vi "ACT_Loop.vi"() -> ()   [LabVIEW 2023, in "Pivot FX_ACT.lvlib"]
uses:
  Pivot FX_ACT.lvlib
  RoboRIO Utilities/Global_STOP.vi
  ENUM_ACT_Action.ctl
  ENUM_ACT_State.ctl
  Global_CMD_ACT_Data In.vi
  Global_ACT_Data Out.vi
  Cluster_CMD_ACT_Data.ctl
  <vilib>/Rock Robotics/WPI/MotorControl/WPI_MotorControlType.ctl
  <vilib>/Rock Robotics/SystemInterfaces/DIO/FPGA_DIOPWMChannel.ctl
  <vilib>/Rock Robotics/WPI/PWM/WPI_PWMDeadband.ctl
  <vilib>/Rock Robotics/SystemInterfaces/DIO/FPGA_DIOChannel.ctl
  <vilib>/Rock Robotics/WPI/MotorControl/WPI_MotorControlDeviceRef.ctl
  Shared Code/TypeDefs/Cluser_CAN Data.ctl
  <vilib>/Rock Robotics/WPI/ThirdParty/Phoenix-LabVIEW/Motor Controller/Controls/CTRE_Phoenix_MotorControl_NeutralMode.ctl
  Shared Code/TypeDefs/Cluster_FWD  REV Values.ctl
  Shared Code/TypeDefs/Cluster_PID Gains.ctl
  Shared Code/TypeDefs/Cluster_FX Motion Magic Parameters.ctl
  <vilib>/Rock Robotics/WPI/ThirdParty/Phoenix-LabVIEW/Motor Controller/Controls/CTRE_Phoenix_MotorControl_LimitSwitchNormal.ctl
  Shared Code/TypeDefs/Cluser_Hard Limits.ctl
  Shared Code/TypeDefs/Cluser_Enable-Value I32.ctl
  Shared Code/TypeDefs/Cluser_Config_Soft Limits.ctl
  Shared Code/TypeDefs/Cluser_FX Config_Limit Travel.ctl
  Cluster_Config HW Values.ctl
  b5508d6c-c1cc-4273-80c5-2077d34e1483.vi
  5f725c2a-0ce1-4524-8967-e83b15fdce90.vi
  <vilib>/Rock Robotics/WPI/ThirdParty/Phoenix-LabVIEW/Motor Controller/Controls/CTRE_Phoenix_MotorControl_ControlMode.ctl
  Shared Code/TypeDefs/Cluster_FX CloseLoop Values.ctl
  Shared Code/TypeDefs/Cluster_FX Current Values.ctl
  Cluster_HW Output Values.ctl
  ENUM_CMD_Mode Select.ctl
  4f1f8321-3dc8-4b28-8619-20673fc77ec2.vi
  Cluster_SW Output Data.ctl
  Cluster_Config SW Values.ctl
  36677ea0-a1a5-47a3-bc56-4475cb7c281e.vi
  573e44c0-11f4-4bd9-ad56-904ec25dba75.vi
  e7494af9-f670-4352-9dfa-ae6ce50709ea.vi
  6201c2b1-dcd8-4430-86f1-9b4ee56c7753.vi
  Shared Code/TypeDefs/Cluser_FX Config_Current Limits.ctl
  Shared Code/TypeDefs/Cluster_FX SLOT PID Config.ctl
  <vilib>/Rock Robotics/WPI/ThirdParty/Phoenix-LabVIEW/Motor Controller/Controls/CTRE_Phoenix_MotorControl_TalonFXInvertType.ctl
  Shared Code/TypeDefs/Cluster_Config FX Motor Output.ctl
  Shared Code/TypeDefs/ENUM_Pivot Arm Position Select.ctl
  Shared Code/TypeDefs/Cluster_Pivot Arm Position Table.ctl
  Shared Code/TypeDefs/Cluster_FX Limit Switchs.ctl
  Shared Code/TypeDefs/Cluster_FX Voltage Values.ctl
  Shared Code/TypeDefs/Cluster_FX Sensor Values.ctl
panel:
  out "STATE":T1
  in  "CMD Override":T2(tab)
  in  "Enable 1":bool
  in  "Percent Out":dbl(slide) scale=-1.0..1.0
  in  "Enable 2":bool
  in  "Position Counts":dbl
  in  "Enable 3":bool
  in  "Position Select":T3
  out "Current Time":timestamp
  in  "SW Config":T4={"Ver"=0, "Pivot Arm Position Table"={"Full Back"=0.0, "Full Forward"=140000.0, "Amp Score"=138000.0, "Pivot Arm Load"=17100.0, "Vertical"=72600.0, "Trap Score"=140000.0}}
  out "SW Output":T6
  out "Sensor Read time":dbl format="%.3g"
  out "HW Sensors":T7
  in  "Read Saved Config":bool
  in  "Update Config":bool
  in  "HW Config":T13 {"CL"."Gains"."F" format="%#.8f"; "CL"."Gains"."D" format="%#.8f"; "CL"."Gains"."I" format="%#.8f"; "CL"."Gains"."P" format="%#.8f"; "Output"."Min"."REV" format="%.2f"; "Output"."Min"."FWD" format="%.2f"; "Output"."Max"."REV" format="%.2f"; "Output"."Max"."FWD" format="%.2f"; "TravelLimits"."Soft"."REV"."Counts" format="%#.0f"; "TravelLimits"."Soft"."FWD"."Counts" format="%#.0f"}
  out "CMD":T28
  out "Cycle Time (S)":dbl format="%.3g"
  # "Teleop - Auto"
  # "STOP"
  # "Tune Output\nto 1023 Max"
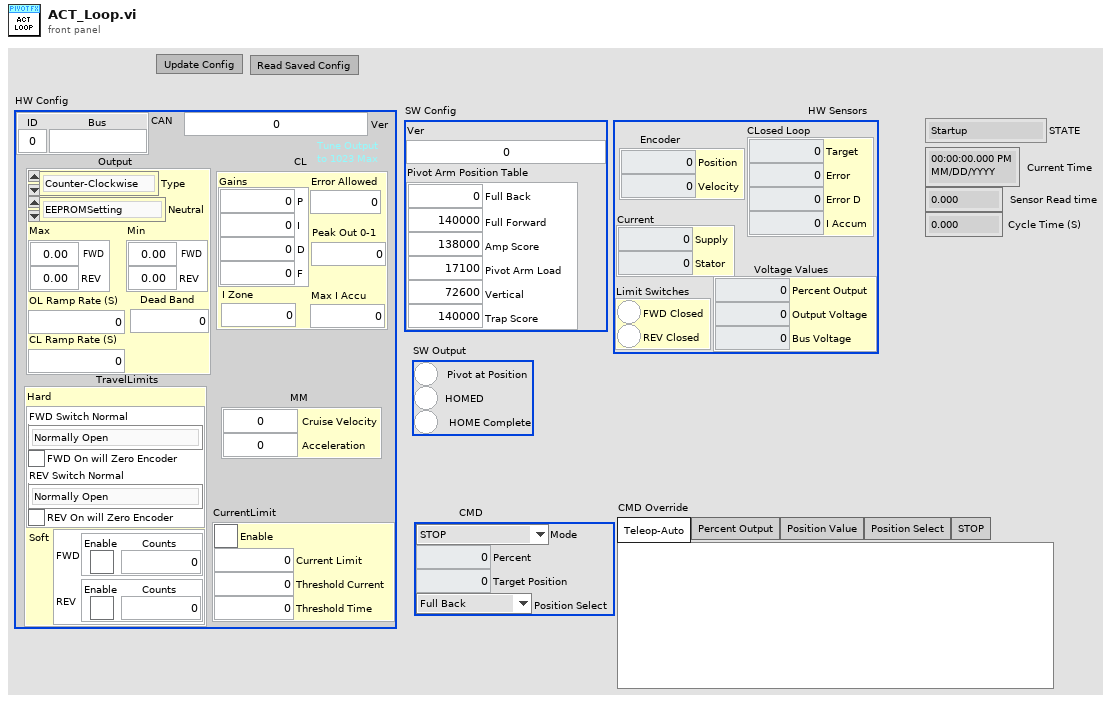
[diagram p1: front panel]
types:
  T1 = typedef "Pivot FX_ACT.lvlib/ENUM_ACT_State.ctl" = enum16{"Startup", "Configuring", "Homming", "Stopping", "Moving Percent Out", "Moving to Position", "Shutdown"}
  T2 = enum32{"Teleop-Auto", "Percent Output", "Position Value", "Position Select", "STOP"}
  T3 = typedef "ENUM_Pivot Arm Position Select.ctl" = enum16{"Full Back", "Full Forward", "Amp Score", "Pivot Arm Load", "Vertical", "Trap Score"}
  T4 = typedef "Pivot FX_ACT.lvlib/Cluster_Config SW Values.ctl" = cluster{"Ver":u64, "Pivot Arm Position Table":T5}
  T5 = typedef "Cluster_Pivot Arm Position Table.ctl" = cluster{"Full Back":dbl, "Full Forward":dbl, "Amp Score":dbl, "Pivot Arm Load":dbl, "Vertical":dbl, "Trap Score":dbl}
  T6 = typedef "Pivot FX_ACT.lvlib/Cluster_SW Output Data.ctl" = cluster{"Pivot at Position":bool, "HOMED":bool, "HOME Complete":bool}
  T7 = typedef "Pivot FX_ACT.lvlib/Cluster_HW Output Values.ctl" = cluster{"CLosed Loop":T8, "Current":T9, "Limit Switches":T10, "Voltage Values":T11, "Encoder ":T12}
  T8 = typedef "Cluster_FX CloseLoop Values.ctl" = cluster{"Target":dbl, "Error":i32, "Error D":dbl, "I Accum":dbl}
  T9 = typedef "Cluster_FX Current Values.ctl" = cluster{"Supply":dbl, "Stator":dbl}
  T10 = typedef "Cluster_FX Limit Switchs.ctl" = cluster{"FWD Closed":bool, "REV Closed":bool}
  T11 = typedef "Cluster_FX Voltage Values.ctl" = cluster{"Percent Output":dbl, "Output Voltage":dbl, "Bus Voltage":dbl}
  T12 = typedef "Cluster_FX Sensor Values.ctl" = cluster{"Position":i32, "Velocity":i32}
  T13 = typedef "Pivot FX_ACT.lvlib/Cluster_Config HW Values.ctl" = cluster{"Ver":u64, "CAN":T14, "Output":T15, "CL":T19, "MM":T21, "TravelLimits":T22, "CurrentLimit":T27}
  T14 = typedef "Cluser_CAN Data.ctl" = cluster{"ID":u8, "Bus":string}
  T15 = typedef "Cluster_Config FX Motor Output.ctl" = cluster{"Type":T16, "Neutral":T17, "Max":T18, "Min":T18, "OL Ramp Rate (S)":dbl, "Dead Band":dbl, "CL Ramp Rate (S)":dbl}
  T16 = typedef "CTRE_Phoenix_MotorControl_TalonFXInvertType.ctl" = enum16{"Counter-Clockwise", "Clockwise"}
  T17 = typedef "CTRE_Phoenix_MotorControl_NeutralMode.ctl" = enum8{"EEPROMSetting", "Override to Coast", "Override to Brake"}
  T18 = typedef "Cluster_FWD  REV Values.ctl" = cluster{"FWD":dbl, "REV":dbl}
  T19 = typedef "Cluster_FX SLOT PID Config.ctl" = cluster{"Gains":T20, "Error Allowed":dbl, "I Zone":dbl, "Peak Out 0-1":dbl, "Max I Accu":dbl}
  T20 = typedef "Cluster_PID Gains.ctl" = cluster{"P":dbl, "I":dbl, "D":dbl, "F":dbl}
  T21 = typedef "Cluster_FX Motion Magic Parameters.ctl" = cluster{"Cruise Velocity":i32, "Acceleration":i32}
  T22 = typedef "Cluser_FX Config_Limit Travel.ctl" = cluster{"Hard":T23, "Soft":T25}
  T23 = typedef "Cluser_Hard Limits.ctl" = cluster{"FWD Switch Normal":T24, "FWD On will Zero Encoder ":bool, "REV Switch Normal":T24, "REV On will Zero Encoder ":bool}
  T24 = typedef "CTRE_Phoenix_MotorControl_LimitSwitchNormal.ctl" = enum16{"Normally Open", "Normally Closed", "Disabled"}
  T25 = typedef "Cluser_Config_Soft Limits.ctl" = cluster{"FWD":T26, "REV":T26}
  T26 = typedef "Cluser_Enable-Value I32.ctl" = cluster{"Enable":bool, "Counts":i32}
  T27 = typedef "Cluser_FX Config_Current Limits.ctl" = cluster{"Enable":bool, "Current Limit":dbl, "Threshold Current":dbl, "Threshold Time":dbl}
  T28 = typedef "Pivot FX_ACT.lvlib/Cluster_CMD_ACT_Data.ctl" = cluster{"Mode":T29, "Percent":dbl, "Target Position":dbl, "Position Select":T3}
  T29 = typedef "Pivot FX_ACT.lvlib/ENUM_CMD_Mode Select.ctl" = enum16{"STOP", "PercentOut", "Positon Value", "Position Select"}
  T30 = typedef "CTRE_Phoenix_MotorControl_ControlMode.ctl" = u16
  T31 = typedef "WPI_MotorControlDeviceRef.ctl" = cluster{"DeviceStatus":errorcluster, "Type":T32, "PWM":cluster{"PWM Channel":T33, "DeadBand":T34}, "CAN":cluster{"Device Number":u8, "SetOutput VI Ref":variant, "GetOutput VI Ref":variant, "Enable VI Ref":variant, "Disable VI Ref":variant, "Data":variant}, "Invert":bool, "DIO PWM":cluster{"PWM \"Enable\" Channel":T33, "DIOChannel":T35, "PWM Rate":dbl}}
  T32 = typedef "WPI_MotorControlType.ctl" = enum16{"PWM", "CAN", "DIO PWM"}
  T33 = typedef "FPGA_DIOPWMChannel.ctl" = enum8{"PWM 0", "PWM 1", "PWM 2", "PWM 3", "PWM 4", "PWM 5", "PWM 6", "PWM 7", "PWM 8", "PWM 9", "PWM MXP 0", "PWM MXP 1", "PWM MXP 2", "PWM MXP 3", "PWM MXP 4", "PWM MXP 5", "PWM MXP 6", "PWM MXP 7", "PWM MXP 8", "PWM MXP 9", "Invalid"}
  T34 = typedef "WPI_PWMDeadband.ctl" = cluster{"Name":string, "maxPositivePwm":i32, "minPositivePwm":i32, "centerPwm":i32, "maxNegativePwm":i32, "minNegativePwm":i32, "angularRange":u16}
  T35 = typedef "FPGA_DIOChannel.ctl" = enum8{"DIO 0", "DIO 1", "DIO 2", "DIO 3", "DIO 4", "DIO 5", "DIO 6", "DIO 7", "DIO 8", "DIO 9", "DIO MXP 0", "DIO MXP 1", "DIO MXP 2", "DIO MXP 3", "DIO MXP 4", "DIO MXP 5", "DIO MXP 6", "DIO MXP 7", "DIO MXP 8", "DIO MXP 9", "DIO MXP 10", "DIO MXP 11", "DIO MXP 12", "DIO MXP 13", "DIO MXP 14", "DIO MXP 15", "SPI Port CS1", "SPI Port CS2", "SPI Port CS3", "SPI Port MISO", "SPI Port MOSI", "Invalid"}
  T36 = cluster{"Team Files Folder":path, "FX Ref":T31, "State":T1, "Previous State":T1, "Current Time":timestamp, "Previous Time":timestamp, "Start Time":timestamp, "Target Time (ms)":u32, "Cycle Time(S)":dbl, "Update Display":bool, "ACT Input":T28, "HW Config":T13, "SW Config":T4, "Max # Of Config Tries":i32, "HW Out":T7, "SW Out":T6, "CAN Timeout":u32, "FX Mode":T30, "FX Set Value":dbl}
  T37 = typedef "Pivot FX_ACT.lvlib/ENUM_ACT_Action.ctl" = enum16{"No Action", "Reset Time", "Reset All", "Config HW File Read", "Config HW File Save", "Config SW File Read", "Config SW File Save", "Config From FP", "Config HW Get", "Config HW Set", "Open HW Only", "Control FX Stop", "Control FX Percent Out", "Control FX Position Value", "Control FX Position Select", "Control FX GoTo HOME", "Encoder Set to Zero"}
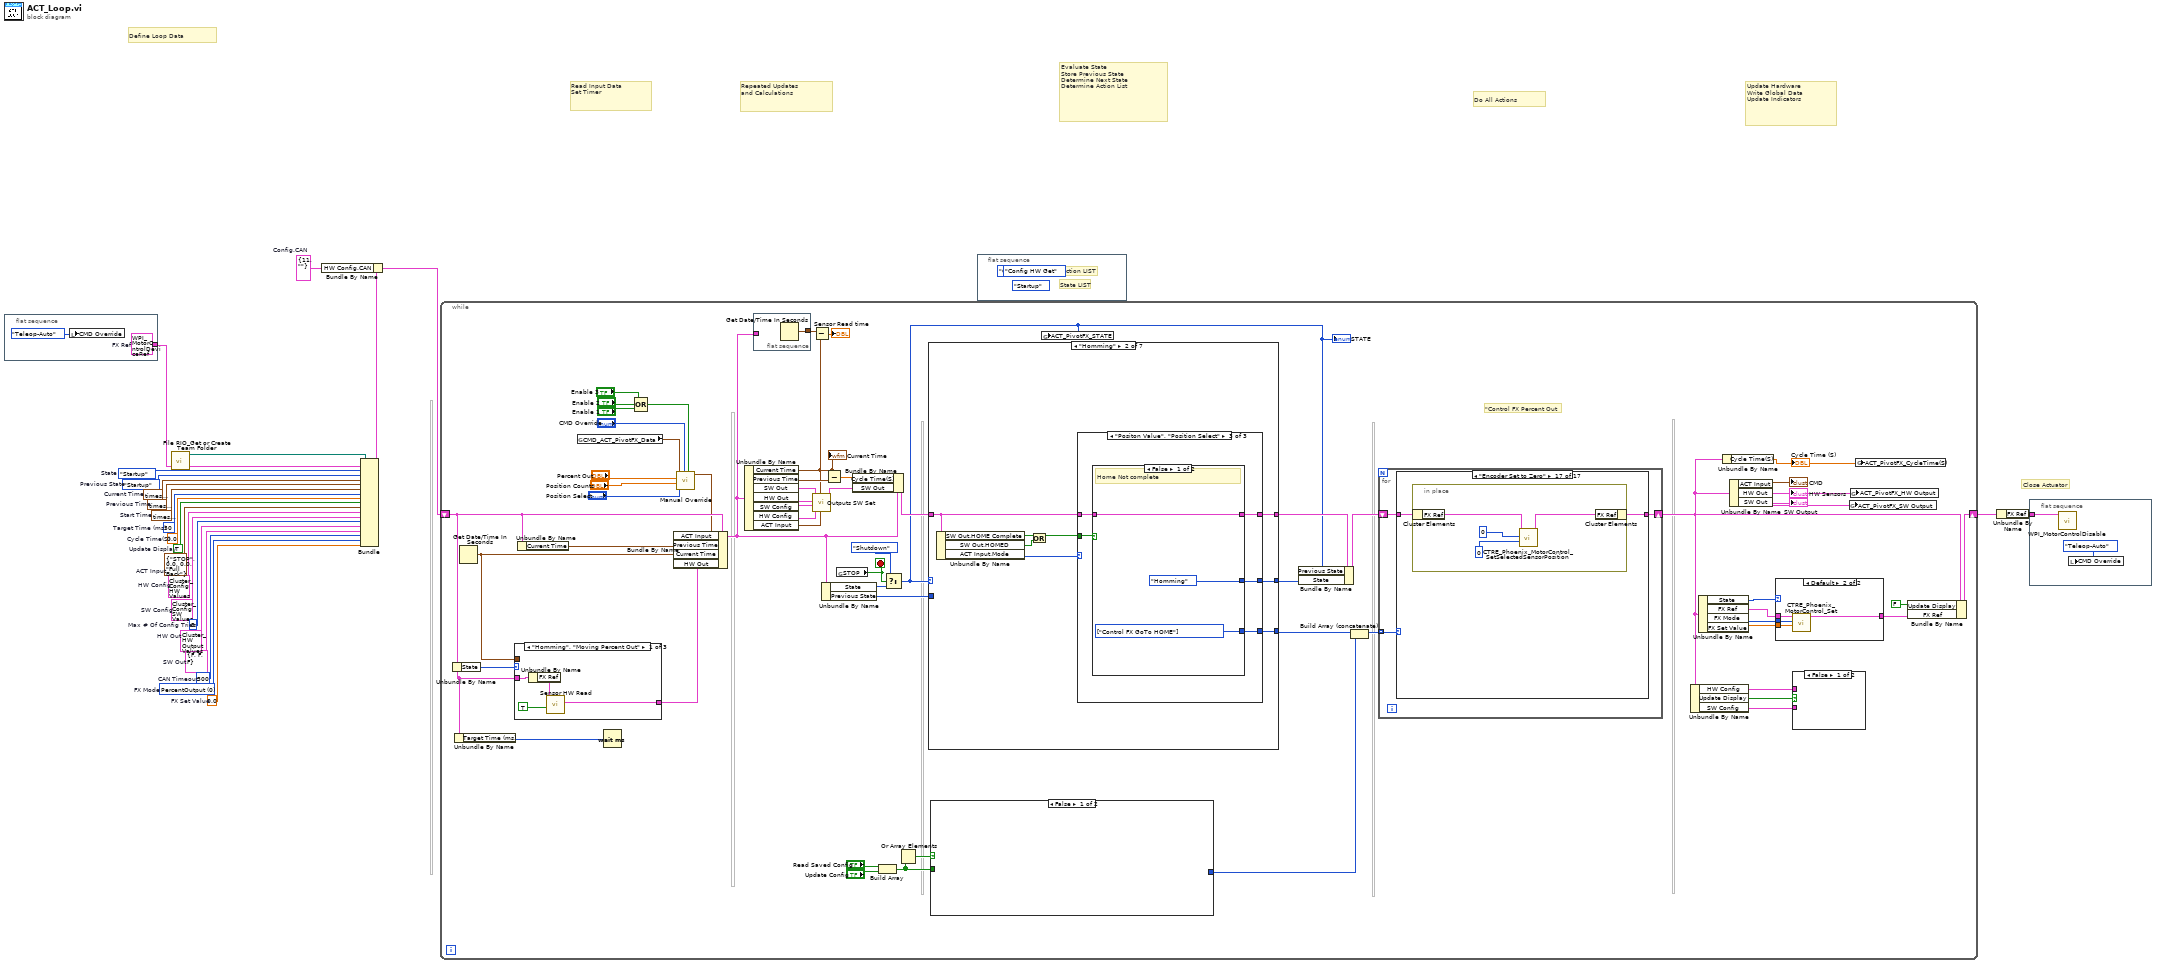
[diagram p0: block diagram]
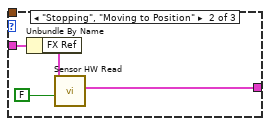
[diagram p2: hidden frame]
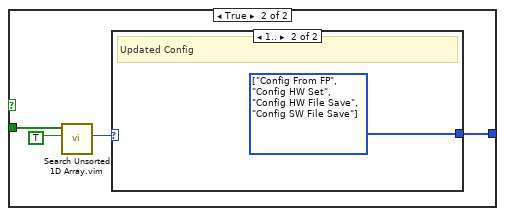
[diagram p4: hidden frame]
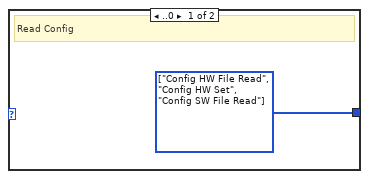
[diagram p5: hidden frame]
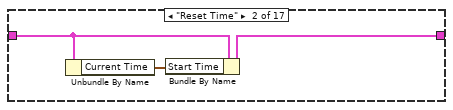
[diagram p7: hidden frame]
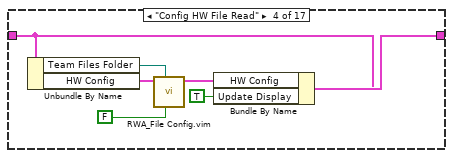
[diagram p9: hidden frame]
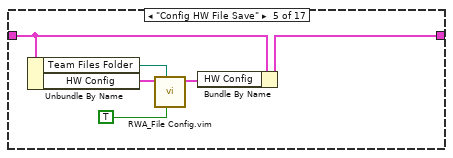
[diagram p10: hidden frame]
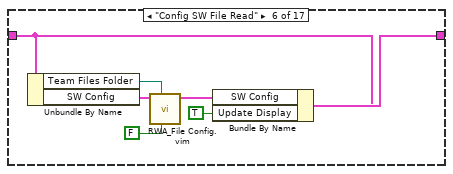
[diagram p11: hidden frame]
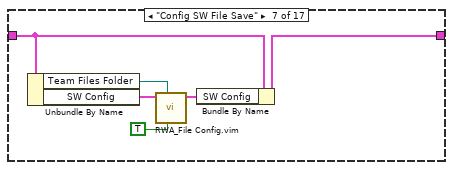
[diagram p12: hidden frame]
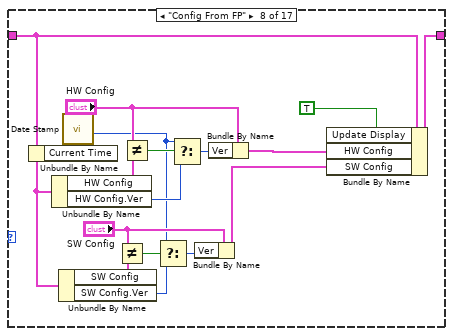
[diagram p13: hidden frame]
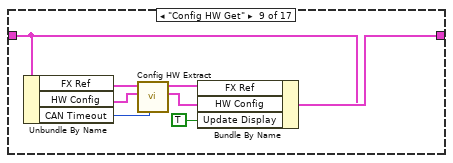
[diagram p14: hidden frame]
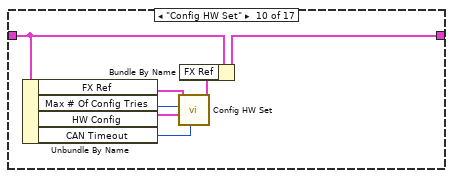
[diagram p15: hidden frame]
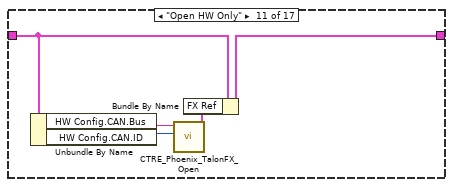
[diagram p16: hidden frame]
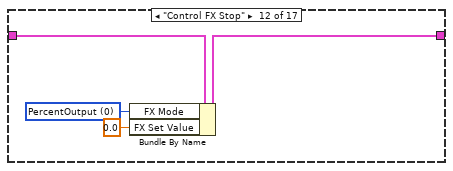
[diagram p17: hidden frame]
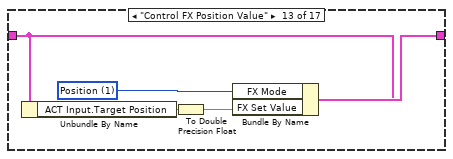
[diagram p18: hidden frame]
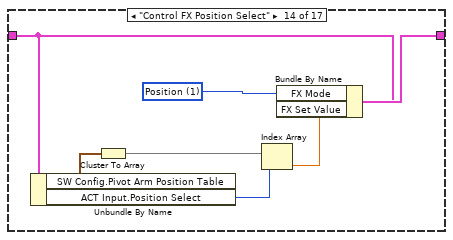
[diagram p19: hidden frame]
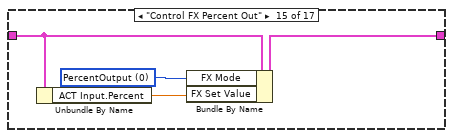
[diagram p20: hidden frame]
diagram:
  w1 = T4 {"Ver"=0, "Pivot Arm Position Table"={"Full Back"=0.0, "Full Forward"=140000.0, "Amp Score"=138473.0, "Pivot Arm Load"=17141.0, "Vertical"=72668.0, "Trap Score"=140000.0}}  # SW Config
  w10 = T13 {"Ver"=0, "CAN"={"ID"=0, "Bus"=""}, "Output"={"Type"=enum."Counter-Clockwise", "Neutral"=enum."EEPROMSetting", "Max"={"FWD"=0.0, "REV"=0.0}, "Min"={"FWD"=0.0, "REV"=0.0}, "OL Ramp Rate (S)"=0.0, "Dead Band"=0.0, "CL Ramp Rate (S)"=0.0}, "CL"={"Gains"={"P"=0.0, "I"=0.0, "D"=0.0, "F"=0.0}, "Error Allowed"=0.0, "I Zone"=0.0, "Peak Out 0-1"=0.0, "Max I Accu"=0.0}, "MM"={"Cruise Velocity"=0, "Acceleration"=0}, "TravelLimits"={"Hard"={"FWD Switch Normal"=enum."Normally Open", "FWD On will Zero Encoder "=FALSE, "REV Switch Normal"=enum."Normally Open", "REV On will Zero Encoder "=FALSE}, "Soft"={"FWD"={"Enable"=FALSE, "Counts"=0}, "REV"={"Enable"=FALSE, "Counts"=0}}}, "CurrentLimit"={"Enable"=FALSE, "Current Limit"=0.0, "Threshold Current"=0.0, "Threshold Time"=0.0}}  # HW Config
  w8 = T6 {"Pivot at Position"=FALSE, "HOMED"=FALSE, "HOME Complete"=FALSE}  # SW Out
  w9 = T7 {"CLosed Loop"={"Target"=0.0, "Error"=0, "Error D"=0.0, "I Accum"=0.0}, "Current"={"Supply"=0.0, "Stator"=0.0}, "Limit Switches"={"FWD Closed"=FALSE, "REV Closed"=FALSE}, "Voltage Values"={"Percent Output"=0.0, "Output Voltage"=0.0, "Bus Voltage"=0.0}, "Encoder "={"Position"=0, "Velocity"=0}}  # HW Out
  w4 = 0.0  # FX Set Value
  w5 = T30 0 items=["PercentOutput"=0, "Position"=1, "Velocity"=2, "Current"=3, "Follower"=5, "MotionProfile"=6, "MotionMagic"=7, "MotionProfileArc"=10, "Disabled"=15]  # FX Mode
  w3 = u32 300  # CAN Timeout
  w2 = 3  # Max # Of Config Tries
  w12 = TRUE  # Update Display
  w13 = T14 {"ID"=11, "Bus"=""}  # Config.CAN
  w18 = 0.0  # Cycle Time(S)
  w19 = ENUM_ACT_State."Startup"  # Previous State
  w20 = timestamp(0 s since 1904-01-01)  # Previous Time
  w21 = u32 50  # Target Time (ms)
  w7 = T28 {"Mode"=enum."STOP", "Percent"=0.0, "Target Position"=0.0, "Position Select"=enum."Full Back"}  # ACT Input
  w22 = timestamp(0 s since 1904-01-01)  # Start Time
  w23 = timestamp(0 s since 1904-01-01)  # Current Time
  w24 = ENUM_ACT_State."Startup"  # State
  # "Close Actuator"
  # "Define Loop Data"
  # "Repeated Updates\nand Calculations"
  # "Read Input Data\nSet Timer"
  # "Evaluate State\nStore Previous State\nDetermine Next State\nDetermine Action List"
  # "Do All Actions"
  # "Update Hardware\nWrite Global Data\nUpdate Indicators"
  n1 = flat-sequence {
    tunnel: [w26] -> w14
    frame #0 {
      w26 = T31 {"DeviceStatus"={"status"=FALSE, "code"=0, "source"=""}, "Type"=enum."PWM", "PWM"={"PWM Channel"=enum."PWM 1", "DeadBand"={"Name"="", "maxPositivePwm"=0, "minPositivePwm"=0, "centerPwm"=0, "maxNegativePwm"=0, "minNegativePwm"=0, "angularRange"=0}}, "CAN"={"Device Number"=0, "SetOutput VI Ref"=variant(enum8{"Percent VBus", "Current", "Speed", "Position", "Voltage"} enum."Percent VBus"), "GetOutput VI Ref"=variant(refnum<k1> refnum), "Enable VI Ref"=variant(dbl 12.0), "Disable VI Ref"=variant(enum8{"Percent VBus", "Speed", "Position", "Slave", "Unchanged / Invalid", "Voltage Compensation", "Current", "Motion Profile"} enum."Percent VBus"), "Data"=variant}, "Invert"=FALSE, "DIO PWM"={"PWM \"Enable\" Channel"=enum."Invalid", "DIOChannel"=enum."Invalid", "PWM Rate"=0.0}}  # FX Ref
      n2 = local write "CMD Override"(T2."Teleop-Auto" ("CMD Override")) -> ()
    }
  }
  n3 = call "File RIO_Get or Create Team Folder.vi"() -> ("Team Files Folder"=w6:path)  [unwired: 10 in, 1 out]
  n4 = Bundle("Team Files Folder"=w6, "FX Ref"=w14, "State"=w24, "Previous State"=w19, "Current Time"=w23, "Previous Time"=w20, "Start Time"=w22, "Target Time (ms)"=w21, "Cycle Time(S)"=w18, "Update Display"=w12, "ACT Input"=w7, "HW Config"=w10, "SW Config"=w1, "Max # Of Config Tries"=w2, "HW Out"=w9, "SW Out"=w8, "CAN Timeout"=w3, "FX Mode"=w5, "FX Set Value"=w4) -> (w16:T36)  [unwired: 1 in]
  n5 = Bundle By Name(cluster=w16, "HW Config.CAN"=w13) -> (w15:T36)
  n6 = while {
    shift-right: [w69] -> w17
    shift-left: w15 -> [w39]
    stop <- w82 stop-if-true
    # "\"Control FX Percent Out"
    n7 = Unbundle By Name(w39) -> ("State"=w59:T1)
    n8 = Unbundle By Name(w39) -> ("Target Time (ms)"=w79:u32)
    n9 = Get Date/Time In Seconds() -> (seconds since 1Jan1904=w55:timestamp)
    n10 = case shown="\"Homming\", \"Moving Percent Out\"" w59 {
      tunnel: w39 -> [w90 w94 _]
      tunnel: w55 -> [_ _ _]
      tunnel: [w87 w91 _] -> w40
      frame "Homming", "Moving Percent Out" {
        n11 = Unbundle By Name(w90) -> ("FX Ref"=w89:T31)
        n12 = call "Sensor HW Read.vi"("Read Closed Loop"=TRUE, "Ref"=w89) -> ("Sensor Values Out"=w87:T7)  [unwired: 7 in, 2 out]
      }
      frame "Stopping", "Moving to Position" {
        n13 = Unbundle By Name(w94) -> ("FX Ref"=w93:T31)
        n14 = call "Sensor HW Read.vi"("Read Closed Loop"=FALSE, "Ref"=w93) -> ("Sensor Values Out"=w91:T7)  [unwired: 7 in, 2 out]
      }
      frame "Startup", "Configuring", "Shutdown" {
      }
    }
    n15 = Unbundle By Name(w39) -> ("Current Time"=w78:timestamp)
    n16 = global read "Global_CMD_ACT_Data In.vi" "CMD_ACT_PivotFX_Data"() -> (w36:T28)
    n17 = Wait (ms)(milliseconds to wait=w79) -> ()  [unwired: 1 out]
    n18 = Compound Arithmetic op=OR("Enable 3", "Enable 2", "Enable 1") -> (w32:bool)
    n19 = call "Manual Override.vi"("Enable"=w32, "CMD Override"="CMD Override", "Pivot Position Select"="Position Select", "Position Data"="Position Counts", "Percent Out Data"="Percent Out", "Auto CMD"=w36) -> ("OverRide Command Out"=w38:T28)  [unwired: 5 in]
    n20 = Bundle By Name(cluster=w39, "ACT Input"=w38, "Previous Time"=w78, "Current Time"=w55, "HW Out"=w40) -> (w41:T36)
    n21 = Unbundle By Name(w41) -> ("Current Time"=w45:timestamp, "Previous Time"=w76:timestamp, "SW Out"=w48:T6, "HW Out"=w46:T7, "SW Config"=w44:T4, "HW Config"=w43:T13, "ACT Input"=w27:T28)
    "Current Time" <- w45
    n22 = flat-sequence {
      tunnel: [w86] -> w57
      tunnel: w41 -> [_]
      frame #0 {
        n23 = Get Date/Time In Seconds() -> (seconds since 1Jan1904=w86:timestamp)
      }
    }
    n24 = call "Outputs SW Set.vi"("CMD_ACT_Tempplate Data"=w27, "Current Time"=w45, "HW Config"=w43, "SW Config"=w44, "Sensor Values"=w46, "SW Output"=w48) -> ("SW Output Out"=w47:T6)  [unwired: 5 in]
    n25 = Subtract(x=w57, y=w45) -> (x-y=→"Sensor Read time":dbl)
    n26 = Unbundle By Name(w41) -> ("State"=w80:T1, "Previous State"=w77:T1)
    n27 = Subtract(x=w45, y=w76) -> (x-y=w74:dbl)
    n28 = global read "Global_STOP.vi" "STOP"() -> (w82:bool)
    n29 = Bundle By Name(cluster=w41, "Cycle Time(S)"=w74, "SW Out"=w47) -> (w75:T36)
    n30 = Build Array("Read Saved Config", "Update Config") -> (w51:bool[])
    n31 = Select(t=ENUM_ACT_State."Shutdown" ("State"), s=w82, f=w80) -> (s? t:f=w37:T1)
    "STATE" <- w37
    n32 = Or Array Elements(Boolean array=w51) -> (logical OR=w52:bool)
    n33 = case shown="\"Homming\"" w37 {
      selector: w37 -> [_ _ w253 w273 _ _ _]
      tunnel: w75 -> [w207 w232 w254 w274 w301 w304 w309]
      tunnel: [w210 w231 w255 w275 w301 w304 w308] -> w84
      tunnel: [w209 w229 w257 w277 ENUM_ACT_State."Shutdown" ("State") ENUM_ACT_State."Configuring" ("State") w307] -> w83
      tunnel: [w208 w230 w252 w271 w299 w303 w305] -> w73
      tunnel: w77 -> [_ _ _ _ _ _ _]
      frame "Configuring" {
        n34 = Unbundle By Name(w207) -> ("SW Config"=w205:T4)
        n35 = Unbundle By Name(w207) -> ("Team Files Folder"=w204:path, "HW Config"=w212:T13)
        n36 = call "Config_Build Name.vim"("Config First Name"=w212) -> ("Cfg file"=w214:string)  [unwired: 9 in, 1 out]
        n37 = call "Config_Build Name.vim"("Config First Name"=w205) -> ("Cfg file"=w206:string)  [unwired: 9 in, 1 out]
        n38 = Build Path(base path=w204, name or relative path=w206) -> (appended path=w203:path)
        n39 = Build Path(base path=w204, name or relative path=w214) -> (appended path=w213:path)
        n40 = call <vilib>:"Check if File or Folder Exists.vi"("path"=w203) -> ("file or folder exists?"=w202:bool)  [unwired: 8 in, 2 out]
        n41 = call <vilib>:"Check if File or Folder Exists.vi"("path"=w213) -> ("file or folder exists?"=w211:bool)  [unwired: 8 in, 2 out]
        n42 = case shown="True" w211 {
          tunnel: w207 -> [w217 w221]
          tunnel: [w217 w221] -> w210
          tunnel: [ENUM_ACT_State."Configuring" ("State") w220] -> w209
          tunnel: [w215 w219] -> w208
          tunnel: w202 -> [_ w218]
          frame False {
            w215 = T37[] [enum."Open HW Only", enum."Config HW Get", enum."Config HW File Save"] items=["No Action", "Reset Time", "Reset All", "Config HW File Read", "Config HW File Save", "Config SW File Read", "Config SW File Save", "Config From FP", "Config HW Get", "Config HW Set", "Open HW Only", "Control FX Stop", "Control FX Percent Out", "Control FX Position Value", "Control FX Position Select", "Control FX GoTo HOME", "Encoder Set to Zero"] ("Actions")
            # "HW Config File Not Found"
          }
          frame True {
            # "HW Config File Found"
            n43 = case shown="True" w218 {
              tunnel: [ENUM_ACT_State."Configuring" ("State") ENUM_ACT_State."Stopping" ("State")] -> w220
              tunnel: [w222 w224] -> w219
              frame False {
                w222 = T37[] [enum."Config SW File Save"] items=["No Action", "Reset Time", "Reset All", "Config HW File Read", "Config HW File Save", "Config SW File Read", "Config SW File Save", "Config From FP", "Config HW Get", "Config HW Set", "Open HW Only", "Control FX Stop", "Control FX Percent Out", "Control FX Position Value", "Control FX Position Select", "Control FX GoTo HOME", "Encoder Set to Zero"] ("Actions")
                # "SW Config File NOT Found"
              }
              frame True {
                w224 = T37[] [enum."Config HW File Read", enum."Config HW Set", enum."Config SW File Read", enum."Reset All", enum."Control FX Stop"] items=["No Action", "Reset Time", "Reset All", "Config HW File Read", "Config HW File Save", "Config SW File Read", "Config SW File Save", "Config From FP", "Config HW Get", "Config HW Set", "Open HW Only", "Control FX Stop", "Control FX Percent Out", "Control FX Position Value", "Control FX Position Select", "Control FX GoTo HOME", "Encoder Set to Zero"] ("Actions")
                # "SW Config File Found"
              }
            }
          }
        }
      }
      frame "Homming" {
        n44 = Unbundle By Name(w232) -> ("SW Out.HOME Complete"=w233:bool, "SW Out.HOMED"=w227:bool, "ACT Input.Mode"=w226:T29)
        n45 = Or(x=w233, y=w227) -> (x .or. y?=w228:bool)
        n46 = case shown="\"Positon Value\", \"Position Select\"" w226 {
          tunnel: w232 -> [w236 w239 w244]
          tunnel: [w236 w239 w243] -> w231
          tunnel: [w234 w237 w242] -> w230
          tunnel: [ENUM_ACT_State."Stopping" ("State") ENUM_ACT_State."Moving Percent Out" ("State") w241] -> w229
          tunnel: w228 -> [_ _ w240]
          frame "STOP" {
            w234 = T37[] [enum."Control FX Stop"] items=["No Action", "Reset Time", "Reset All", "Config HW File Read", "Config HW File Save", "Config SW File Read", "Config SW File Save", "Config From FP", "Config HW Get", "Config HW Set", "Open HW Only", "Control FX Stop", "Control FX Percent Out", "Control FX Position Value", "Control FX Position Select", "Control FX GoTo HOME", "Encoder Set to Zero"] ("Actions")
          }
          frame "PercentOut" {
            w237 = T37[] [enum."Control FX Stop"] items=["No Action", "Reset Time", "Reset All", "Config HW File Read", "Config HW File Save", "Config SW File Read", "Config SW File Save", "Config From FP", "Config HW Get", "Config HW Set", "Open HW Only", "Control FX Stop", "Control FX Percent Out", "Control FX Position Value", "Control FX Position Select", "Control FX GoTo HOME", "Encoder Set to Zero"] ("Actions")
          }
          frame "Positon Value", "Position Select" {
            n47 = case shown="False" w240 {
              tunnel: w244 -> [w247 w248]
              tunnel: [w247 w248] -> w243
              tunnel: [w245 w250] -> w242
              tunnel: [ENUM_ACT_State."Homming" ("State") ENUM_ACT_State."Stopping" ("State")] -> w241
              frame False {
                w245 = T37[] [enum."Control FX GoTo HOME"] items=["No Action", "Reset Time", "Reset All", "Config HW File Read", "Config HW File Save", "Config SW File Read", "Config SW File Save", "Config From FP", "Config HW Get", "Config HW Set", "Open HW Only", "Control FX Stop", "Control FX Percent Out", "Control FX Position Value", "Control FX Position Select", "Control FX GoTo HOME", "Encoder Set to Zero"] ("Actions")
                # "Home Not complete"
              }
              frame True {
                w250 = T37[] [enum."Control FX Stop", enum."Encoder Set to Zero"] items=["No Action", "Reset Time", "Reset All", "Config HW File Read", "Config HW File Save", "Config SW File Read", "Config SW File Save", "Config From FP", "Config HW Get", "Config HW Set", "Open HW Only", "Control FX Stop", "Control FX Percent Out", "Control FX Position Value", "Control FX Position Select", "Control FX GoTo HOME", "Encoder Set to Zero"] ("Actions")
                # "Home Complete"
              }
            }
          }
        }
      }
      frame "Moving Percent Out" {
        w251 = T37[] [enum."Control FX Stop"] items=["No Action", "Reset Time", "Reset All", "Config HW File Read", "Config HW File Save", "Config SW File Read", "Config SW File Save", "Config From FP", "Config HW Get", "Config HW Set", "Open HW Only", "Control FX Stop", "Control FX Percent Out", "Control FX Position Value", "Control FX Position Select", "Control FX GoTo HOME", "Encoder Set to Zero"] ("Actions")
        n48 = Unbundle By Name(w254) -> ("ACT Input.Mode"=w256:T29)
        n49 = case shown="\"Position Select\"" w256 {
          tunnel: [ENUM_ACT_State."Stopping" ("State") ENUM_ACT_State."Moving to Position" ("State") ENUM_ACT_State."Moving to Position" ("State") w268] -> w257
          tunnel: w254 -> [w260 w263 w266 w269]
          tunnel: [w260 w263 w266 w269] -> w255
          tunnel: w253 -> [_ _ _ w268]
          tunnel: [w258 w261 w264 w267] -> w252
          tunnel: w251 -> [w258 w261 w264 _]
          frame "STOP" {
          }
          frame "Positon Value" {
          }
          frame "Position Select" {
          }
          frame "PercentOut" {
            w267 = T37[] [enum."Control FX Percent Out"] items=["No Action", "Reset Time", "Reset All", "Config HW File Read", "Config HW File Save", "Config SW File Read", "Config SW File Save", "Config From FP", "Config HW Get", "Config HW Set", "Open HW Only", "Control FX Stop", "Control FX Percent Out", "Control FX Position Value", "Control FX Position Select", "Control FX GoTo HOME", "Encoder Set to Zero"] ("Actions")
          }
        }
      }
      frame "Moving to Position" {
        w272 = T37[] [enum."Control FX Stop"] items=["No Action", "Reset Time", "Reset All", "Config HW File Read", "Config HW File Save", "Config SW File Read", "Config SW File Save", "Config From FP", "Config HW Get", "Config HW Set", "Open HW Only", "Control FX Stop", "Control FX Percent Out", "Control FX Position Value", "Control FX Position Select", "Control FX GoTo HOME", "Encoder Set to Zero"] ("Actions")
        n50 = Unbundle By Name(w274) -> ("SW Out.HOME Complete"=w270:bool, "ACT Input.Mode"=w276:T29)
        n51 = case shown="True" w270 {
          tunnel: [ENUM_ACT_State."Homming" ("State") w286] -> w277
          tunnel: w276 -> [_ w285]
          tunnel: [w279 w284] -> w275
          tunnel: w274 -> [w279 w283]
          tunnel: w273 -> [_ w282]
          tunnel: w272 -> [_ w281]
          tunnel: [_ w280] -> w271
          frame False {
            # "Home Not Complete"
          }
          frame True {
            # "Home Complete"
            n52 = case shown="\"Positon Value\"" w285 {
              tunnel: [ENUM_ACT_State."Stopping" ("State") w290 w294 ENUM_ACT_State."Moving Percent Out" ("State")] -> w286
              tunnel: w283 -> [w289 w292 w293 w298]
              tunnel: [w289 w292 w293 w298] -> w284
              tunnel: w282 -> [_ w290 w294 _]
              tunnel: [w287 w291 w295 w296] -> w280
              tunnel: w281 -> [w287 _ _ w296]
              frame "STOP" {
              }
              frame "Positon Value" {
                w291 = T37[] [enum."Control FX Position Value"] items=["No Action", "Reset Time", "Reset All", "Config HW File Read", "Config HW File Save", "Config SW File Read", "Config SW File Save", "Config From FP", "Config HW Get", "Config HW Set", "Open HW Only", "Control FX Stop", "Control FX Percent Out", "Control FX Position Value", "Control FX Position Select", "Control FX GoTo HOME", "Encoder Set to Zero"] ("Actions")
              }
              frame "Position Select" {
                w295 = T37[] [enum."Control FX Position Select"] items=["No Action", "Reset Time", "Reset All", "Config HW File Read", "Config HW File Save", "Config SW File Read", "Config SW File Save", "Config From FP", "Config HW Get", "Config HW Set", "Open HW Only", "Control FX Stop", "Control FX Percent Out", "Control FX Position Value", "Control FX Position Select", "Control FX GoTo HOME", "Encoder Set to Zero"] ("Actions")
              }
              frame "PercentOut" {
              }
            }
          }
        }
      }
      frame "Shutdown" {
        w299 = T37[] [enum."Reset All"] items=["No Action", "Reset Time", "Reset All", "Config HW File Read", "Config HW File Save", "Config SW File Read", "Config SW File Save", "Config From FP", "Config HW Get", "Config HW Set", "Open HW Only", "Control FX Stop", "Control FX Percent Out", "Control FX Position Value", "Control FX Position Select", "Control FX GoTo HOME", "Encoder Set to Zero"] ("Actions")
      }
      frame "Startup" {
        w303 = T37[] [enum."Reset Time"] items=["No Action", "Reset Time", "Reset All", "Config HW File Read", "Config HW File Save", "Config SW File Read", "Config SW File Save", "Config From FP", "Config HW Get", "Config HW Set", "Open HW Only", "Control FX Stop", "Control FX Percent Out", "Control FX Position Value", "Control FX Position Select", "Control FX GoTo HOME", "Encoder Set to Zero"] ("Actions")
      }
      frame "Stopping" {
        (unwired) TRUE
        w306 = T37[] [enum."Control FX Stop"] items=["No Action", "Reset Time", "Reset All", "Config HW File Read", "Config HW File Save", "Config SW File Read", "Config SW File Save", "Config From FP", "Config HW Get", "Config HW Set", "Open HW Only", "Control FX Stop", "Control FX Percent Out", "Control FX Position Value", "Control FX Position Select", "Control FX GoTo HOME", "Encoder Set to Zero"] ("Actions")
        n53 = Unbundle By Name(w309) -> ("ACT Input.Mode"=w310:T29)
        n54 = case shown="\"Position Select\"" w310 {
          tunnel: w309 -> [w313 w316 w319 w322]
          tunnel: [w313 w316 w319 w322] -> w308
          tunnel: [ENUM_ACT_State."Stopping" ("State") ENUM_ACT_State."Moving Percent Out" ("State") ENUM_ACT_State."Moving to Position" ("State") ENUM_ACT_State."Moving to Position" ("State")] -> w307
          tunnel: [w311 w314 w317 w320] -> w305
          tunnel: w306 -> [w311 w314 w317 w320]
          frame "STOP" {
          }
          frame "PercentOut" {
          }
          frame "Positon Value" {
          }
          frame "Position Select" {
          }
        }
      }
    }
    n55 = case shown="False" w52 {
      tunnel: w51 -> [_ w97]
      tunnel: [_ w95] -> w50
      frame False {
      }
      frame True {
        n56 = call "Search Unsorted 1D Array.vim"("element"=TRUE, "unsorted 1D array"=w97) -> ("index of element"=w96:i32)  [unwired: 9 in]
        n57 = case shown="1.." w96 {
          tunnel: [w99 w100] -> w95
          frame ..0 {
            w99 = T37[] [enum."Config HW File Read", enum."Config HW Set", enum."Config SW File Read"] items=["No Action", "Reset Time", "Reset All", "Config HW File Read", "Config HW File Save", "Config SW File Read", "Config SW File Save", "Config From FP", "Config HW Get", "Config HW Set", "Open HW Only", "Control FX Stop", "Control FX Percent Out", "Control FX Position Value", "Control FX Position Select", "Control FX GoTo HOME", "Encoder Set to Zero"] ("Actions")
            # "Read Config"
          }
          frame 1.. {
            w100 = T37[] [enum."Config From FP", enum."Config HW Set", enum."Config HW File Save", enum."Config SW File Save"] items=["No Action", "Reset Time", "Reset All", "Config HW File Read", "Config HW File Save", "Config SW File Read", "Config SW File Save", "Config From FP", "Config HW Get", "Config HW Set", "Open HW Only", "Control FX Stop", "Control FX Percent Out", "Control FX Position Value", "Control FX Position Select", "Control FX GoTo HOME", "Encoder Set to Zero"] ("Actions")
            # "Updated Config"
          }
        }
      }
    }
    n58 = global write "Global_ACT_Data Out.vi" "ACT_PivotFX_STATE"(w37) -> ()
    n59 = Bundle By Name(cluster=w84, "Previous State"=w37, "State"=w83) -> (w85:T36)
    n60 = Build Array (concatenate)(w73, w50) -> (w67:T37[])
    n61 = for {
      tunnel: w67 -> [w103] mode=indexing
      shift-right: [w102] -> w66
      shift-left: w85 -> [w101]
      n62 = case shown="\"Encoder Set to Zero\"" w103 {
        tunnel: w101 -> [w104 w107 w108 w114 w120 w127 w133 w141 w156 w164 w168 w174 w178 w185 w189 w193 w197]
        tunnel: [w104 w106 w108 w115 w121 w128 w134 w151 w157 w165 w169 w175 w180 w187 w191 w195 w196] -> w102
        frame "No Action" {
        }
        frame "Reset Time" {
          n63 = Unbundle By Name(w107) -> ("Current Time"=w105:timestamp)
          n64 = Bundle By Name(cluster=w107, "Start Time"=w105) -> (w106:T36)
        }
        frame "Reset All" {
        }
        frame "Config HW File Read" {
          n65 = Unbundle By Name(w114) -> ("Team Files Folder"=w111:path, "HW Config"=w113:T13)
          n66 = call "RWA_File Config.vim"("Read(f) Save(t)"=FALSE ("Read(f) Write(t)"), "Target Folder Folder"=w111, "Any Config"=w113) -> ("Any Config Out"=w112:T13)  [unwired: 4 in, 4 out]
          n67 = Bundle By Name(cluster=w114, "HW Config"=w112, "Update Display"=TRUE) -> (w115:T36)
        }
        frame "Config HW File Save" {
          n68 = Unbundle By Name(w120) -> ("Team Files Folder"=w117:path, "HW Config"=w119:T13)
          n69 = call "RWA_File Config.vim"("Read(f) Save(t)"=TRUE ("Read(f) Write(t)"), "Target Folder Folder"=w117, "Any Config"=w119) -> ("Any Config Out"=w118:T13)  [unwired: 4 in, 4 out]
          n70 = Bundle By Name(cluster=w120, "HW Config"=w118) -> (w121:T36)
        }
        frame "Config SW File Read" {
          n71 = Unbundle By Name(w127) -> ("Team Files Folder"=w124:path, "SW Config"=w126:T4)
          n72 = call "RWA_File Config.vim"("Read(f) Save(t)"=FALSE ("Read(f) Write(t)"), "Target Folder Folder"=w124, "Any Config"=w126) -> ("Any Config Out"=w125:T4)  [unwired: 4 in, 4 out]
          n73 = Bundle By Name(cluster=w127, "SW Config"=w125, "Update Display"=TRUE) -> (w128:T36)
        }
        frame "Config SW File Save" {
          n74 = Unbundle By Name(w133) -> ("Team Files Folder"=w130:path, "SW Config"=w132:T4)
          n75 = call "RWA_File Config.vim"("Read(f) Save(t)"=TRUE ("Read(f) Write(t)"), "Target Folder Folder"=w130, "Any Config"=w132) -> ("Any Config Out"=w131:T4)  [unwired: 4 in, 4 out]
          n76 = Bundle By Name(cluster=w133, "SW Config"=w131) -> (w134:T36)
        }
        frame "Config From FP" {
          n77 = Unbundle By Name(w141) -> ("Current Time"=w150:timestamp)
          n78 = Unbundle By Name(w141) -> ("HW Config"=w140:T13, "HW Config.Ver"=w137:u64)
          n79 = Unbundle By Name(w141) -> ("SW Config"=w143:T4, "SW Config.Ver"=w145:u64)
          n80 = call "Date Stamp.vi"("Time"=w150) -> ("U64 Out"=w136:u64)  [unwired: 5 in, 1 out]
          n81 = Not Equal?(x=w143, y="SW Config") -> (x != y?=w146:bool)
          n82 = Not Equal?(x="HW Config", y=w140) -> (x != y?=w138:bool)
          n83 = Select(t=w136, s=w146, f=w145) -> (s? t:f=w144:u64)
          n84 = Select(t=w136, s=w138, f=w137) -> (s? t:f=w135:u64)
          n85 = Bundle By Name(cluster="SW Config", "Ver"=w144) -> (w148:T4)
          n86 = Bundle By Name(cluster="HW Config", "Ver"=w135) -> (w149:T13)
          n87 = Bundle By Name(cluster=w141, "Update Display"=TRUE, "HW Config"=w149, "SW Config"=w148) -> (w151:T36)
        }
        frame "Config HW Get" {
          n88 = Unbundle By Name(w156) -> ("FX Ref"=w159:T31, "HW Config"=w158:T13, "CAN Timeout"=w152:u32)
          n89 = call "Config HW Extract.vi"("Send Cmd Timout(ms)"=w152, "Wrist Config"=w158, "DevRef"=w159) -> ("Wrist Config Data Out"=w154:T13, "DevRef Out"=w155:T31)  [unwired: 6 in, 1 out]
          n90 = Bundle By Name(cluster=w156, "FX Ref"=w155, "HW Config"=w154, "Update Display"=TRUE) -> (w157:T36)
        }
        frame "Config HW Set" {
          n91 = Unbundle By Name(w164) -> ("FX Ref"=w166:T31, "Max # Of Config Tries"=w160:i32, "HW Config"=w162:T13, "CAN Timeout"=w161:u32)
          n92 = call "Config HW Set.vi"("Send Cmd Timout(ms)"=w161, "Wrist Config"=w162, "Max # Of Tries"=w160, "DevRef"=w166) -> ("DevRef Out Out"=w163:T31)  [unwired: 6 in, 1 out]
          n93 = Bundle By Name(cluster=w164, "FX Ref"=w163) -> (w165:T36)
        }
        frame "Open HW Only" {
          n94 = Unbundle By Name(w168) -> ("HW Config.CAN.Bus"=w167:string, "HW Config.CAN.ID"=w171:u8)
          n95 = call <vilib>:"CTRE_Phoenix_TalonFX_Open.vi"("Device Number"=w171, "CAN Bus"=w167) -> ("PhoenixMotorControlDevRef"=w170:T31)  [unwired: 8 in, 1 out]
          n96 = Bundle By Name(cluster=w168, "FX Ref"=w170) -> (w169:T36)
        }
        frame "Control FX Stop" {
          w173 = T30 0 items=["PercentOutput"=0, "Position"=1, "Velocity"=2, "Current"=3, "Follower"=5, "MotionProfile"=6, "MotionMagic"=7, "MotionProfileArc"=10, "Disabled"=15] ("FX Mode")
          n97 = Bundle By Name(cluster=w174, "FX Mode"=w173, "FX Set Value"=0.0) -> (w175:T36)
        }
        frame "Control FX Position Value" {
          w179 = T30 1 items=["PercentOutput"=0, "Position"=1, "Velocity"=2, "Current"=3, "Follower"=5, "MotionProfile"=6, "MotionMagic"=7, "MotionProfileArc"=10, "Disabled"=15] ("FX Mode")
          n98 = Unbundle By Name(w178) -> ("ACT Input.Target Position"=w176:dbl)
          n99 = To Double Precision Float(number=w176) -> (double precision float=w177:dbl)
          n100 = Bundle By Name(cluster=w178, "FX Mode"=w179, "FX Set Value"=w177) -> (w180:T36)
        }
        frame "Control FX Position Select" {
          w186 = T30 1 items=["PercentOutput"=0, "Position"=1, "Velocity"=2, "Current"=3, "Follower"=5, "MotionProfile"=6, "MotionMagic"=7, "MotionProfileArc"=10, "Disabled"=15] ("FX Mode")
          n101 = Unbundle By Name(w185) -> ("SW Config.Pivot Arm Position Table"=w184:T5, "ACT Input.Position Select"=w182:T3)
          n102 = Cluster To Array(cluster=w184) -> (array=w183:dbl[])
          n103 = Index Array(array=w183, index=w182) -> (element=w181:dbl)
          n104 = Bundle By Name(cluster=w185, "FX Mode"=w186, "FX Set Value"=w181) -> (w187:T36)
        }
        frame "Control FX Percent Out" {
          w190 = T30 0 items=["PercentOutput"=0, "Position"=1, "Velocity"=2, "Current"=3, "Follower"=5, "MotionProfile"=6, "MotionMagic"=7, "MotionProfileArc"=10, "Disabled"=15] ("FX Mode")
          n105 = Unbundle By Name(w189) -> ("ACT Input.Percent"=w188:dbl)
          n106 = Bundle By Name(cluster=w189, "FX Mode"=w190, "FX Set Value"=w188) -> (w191:T36)
        }
        frame "Control FX GoTo HOME" {
          w194 = T30 0 items=["PercentOutput"=0, "Position"=1, "Velocity"=2, "Current"=3, "Follower"=5, "MotionProfile"=6, "MotionMagic"=7, "MotionProfileArc"=10, "Disabled"=15] ("FX Mode")
          n107 = Bundle By Name(cluster=w193, "FX Mode"=w194, "FX Set Value"=-0.2 ("HW Out.Set.Value")) -> (w195:T36)
        }
        frame "Encoder Set to Zero" {
          n108 = in-place {
            n109 = in-place-cluster #1(w197) -> ("FX Ref"=w201:T31)
            n110 = call <vilib>:"CTRE_Phoenix_MotorControl_SetSelectedSensorPosition.vi"("pidLoopIdx"=u32 0, "New Sensor Position"=0, "PhoenixMotorControlDevRef"=w201) -> ("PhoenixMotorControlDevRef"=w200:T31)  [unwired: 7 in, 1 out]
            n111 = in-place-cluster #1("FX Ref"=w200) -> (w196:T36)
          }
        }
      }
    }
    n112 = Unbundle By Name(w66) -> ("HW Config"=w63:T13, "Update Display"=w64:bool, "SW Config"=w42:T4)
    n113 = Unbundle By Name(w66) -> ("State"=w60:T1, "FX Ref"=w71:T31, "FX Mode"=w61:T30, "FX Set Value"=w62:dbl)
    n114 = Unbundle By Name(w66) -> ("Cycle Time(S)"=w68:dbl)
    "Cycle Time (S)" <- w68
    n115 = Unbundle By Name(w66) -> ("ACT Input"=→"CMD":T28, "HW Out"=w58:T7, "SW Out"=w49:T6)
    "HW Sensors" <- w58
    "SW Output" <- w49
    n116 = case shown="Default" w60 {
      tunnel: w71 -> [w323 w327]
      tunnel: [w323 w326] -> w70
      tunnel: w62 -> [_ w325]
      tunnel: w61 -> [_ w324]
      frame "Startup", "Configuring" {
      }
      frame Default {
        n117 = call <vilib>:"CTRE_Phoenix_MotorControl_Set.vi"("Output"=w325, "Control Mode"=w324, "PhoenixMotorControlDevRef"=w327) -> ("PhoenixMotorControlDevRef"=w326:T31)  [unwired: 7 in, 1 out]
      }
    }
    n118 = case shown="False" w64 {
      tunnel: w63 -> [_ w329]
      tunnel: w42 -> [_ w328]
      frame False {
      }
      frame True {
        n119 = local write "SW Config"(w328) -> ()
        n120 = local write "HW Config"(w329) -> ()
      }
    }
    n121 = global write "Global_ACT_Data Out.vi" "ACT_PivotFX_SW Output"(w49) -> ()
    n122 = global write "Global_ACT_Data Out.vi" "ACT_PivotFX_HW Output"(w58) -> ()
    n123 = global write "Global_ACT_Data Out.vi" "ACT_PivotFX_CycleTime(S)"(w68) -> ()
    n124 = Bundle By Name(cluster=w66, "Update Display"=FALSE, "FX Ref"=w70) -> (w69:T36)
  }
  n125 = flat-sequence {
    frame #0 {
      (unwired) ENUM_ACT_Action."Open HW Only" ("Action")
      (unwired) ENUM_ACT_State."Startup" ("State")
      (unwired) ENUM_ACT_Action."Config HW Get" ("Action")
      # "State LIST"
      # "Action LIST"
    }
  }
  n126 = Unbundle By Name(w17) -> ("FX Ref"=w11:T31)
  n127 = flat-sequence {
    tunnel: w11 -> [w331]
    frame #0 {
      n128 = call <vilib>:"WPI_MotorControlDisable.vi"("MotorControlDevRef"=w331) -> ()  [unwired: 9 in, 2 out]
      n129 = local write "CMD Override"(T2."Teleop-Auto" ("CMD Override")) -> ()
    }
  }
